vi "Sort References By Type.vi"(10 "Controls[]":refnum<vi>[](array[refnum])) -> (2 "Controls":T1)   [LabVIEW 2015, in "AutoRegistration.lvlib" / "AbstractAutoRegistration.lvclass"]
uses:
  AbstractAutoRegistration.lvclass
  Registration References.ctl
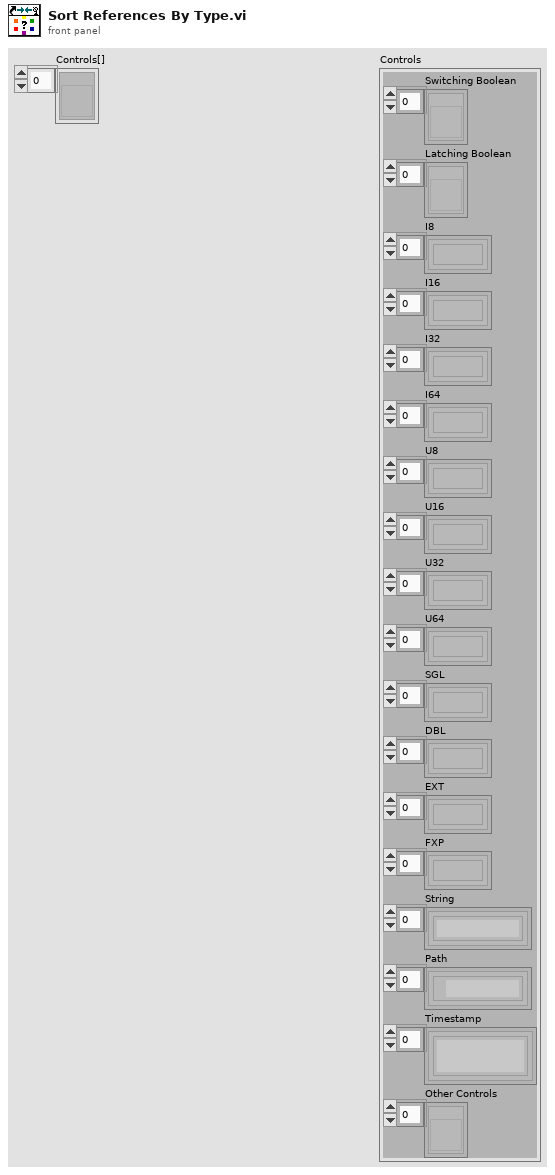
[diagram p1: front panel]
types:
  T1 = typedef "AutoRegistration.lvlib/AbstractAutoRegistration.lvclass/Registration References.ctl" = cluster{"Switching Boolean":refnum<vi>[], "Latching Boolean":refnum<vi>[], "I8":refnum<vi>[], "I16":refnum<vi>[], "I32":refnum<vi>[], "I64":refnum<vi>[], "U8":refnum<vi>[], "U16":refnum<vi>[], "U32":refnum<vi>[], "U64":refnum<vi>[], "SGL":refnum<vi>[], "DBL":refnum<vi>[], "EXT":refnum<vi>[], "FXP":refnum<vi>[], "String":refnum<vi>[], "Path":refnum<vi>[], "Timestamp":refnum<vi>[], "Other Controls":refnum<vi>[]}
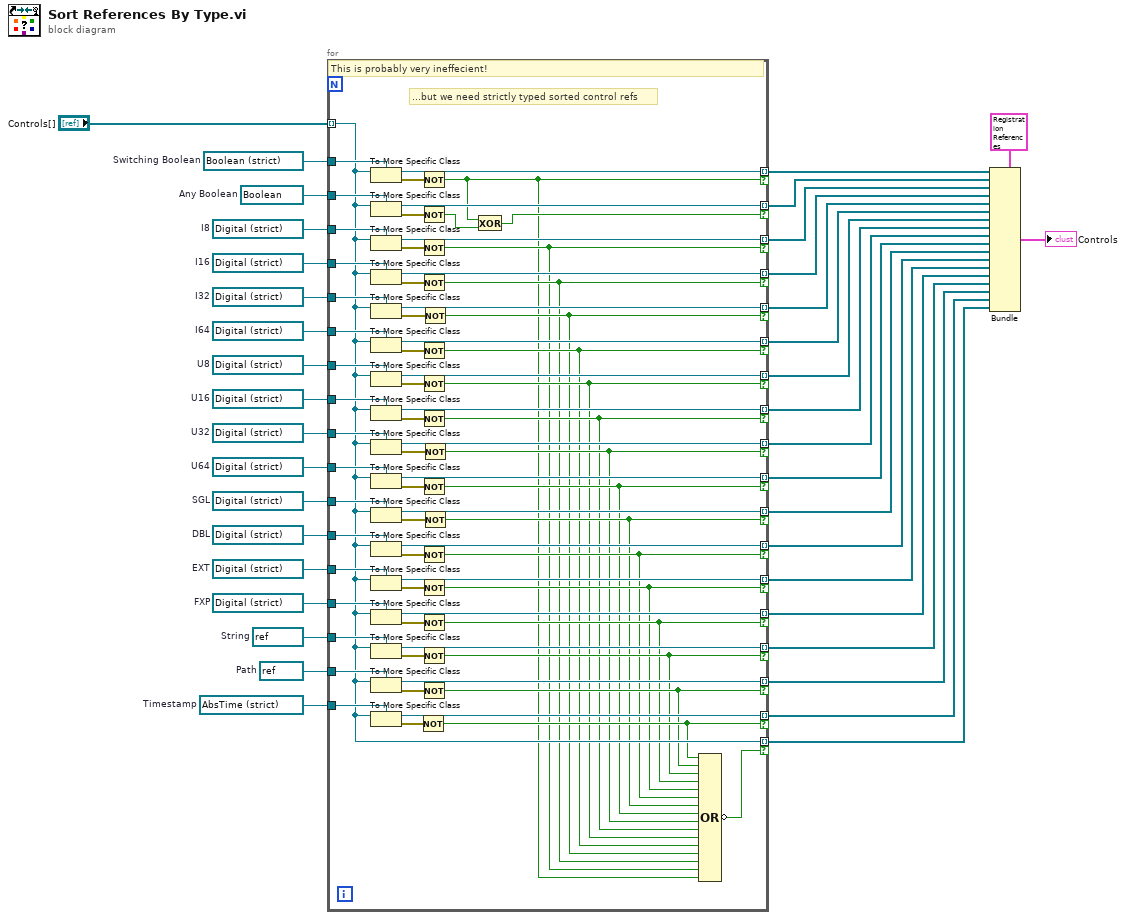
[diagram p0: block diagram]
diagram:
  w21 = refnum<vi> refnum  # Switching Boolean
  w22 = refnum<vi> refnum  # Any Boolean
  w23 = refnum<vi> refnum  # I8
  w24 = refnum<vi> refnum  # I16
  w25 = refnum<vi> refnum  # I32
  w26 = refnum<vi> refnum  # I64
  w27 = refnum<vi> refnum  # U8
  w28 = refnum<vi> refnum  # U16
  w29 = refnum<vi> refnum  # U32
  w30 = refnum<vi> refnum  # U64
  w31 = refnum<vi> refnum  # SGL
  w32 = refnum<vi> refnum  # DBL
  w33 = refnum<vi> refnum  # EXT
  w34 = refnum<vi> refnum  # FXP
  w35 = refnum<vi> refnum  # String
  w36 = refnum<vi> refnum  # Path
  w37 = refnum<vi> refnum  # Timestamp
  n1 = for {
    tunnel: "Controls[]" -> [w56] mode=indexing
    tunnel: w37 -> [w109]
    tunnel: w36 -> [w108]
    tunnel: w35 -> [w107]
    tunnel: w34 -> [w106]
    tunnel: w33 -> [w105]
    tunnel: w32 -> [w104]
    tunnel: w31 -> [w103]
    tunnel: w30 -> [w102]
    tunnel: w29 -> [w101]
    tunnel: w28 -> [w100]
    tunnel: w27 -> [w99]
    tunnel: w26 -> [w98]
    tunnel: w25 -> [w97]
    tunnel: w24 -> [w96]
    tunnel: w23 -> [w95]
    tunnel: w22 -> [w94]
    tunnel: w21 -> [w93]
    tunnel: [w92] -> w20 mode=indexing if=w39
    tunnel: [w91] -> w19 mode=indexing if=w57
    tunnel: [w90] -> w18 mode=indexing if=w40
    tunnel: [w89] -> w17 mode=indexing if=w41
    tunnel: [w88] -> w16 mode=indexing if=w42
    tunnel: [w87] -> w15 mode=indexing if=w43
    tunnel: [w86] -> w14 mode=indexing if=w44
    tunnel: [w85] -> w13 mode=indexing if=w45
    tunnel: [w84] -> w12 mode=indexing if=w46
    tunnel: [w83] -> w11 mode=indexing if=w47
    tunnel: [w82] -> w10 mode=indexing if=w48
    tunnel: [w81] -> w9 mode=indexing if=w49
    tunnel: [w80] -> w8 mode=indexing if=w50
    tunnel: [w79] -> w7 mode=indexing if=w51
    tunnel: [w78] -> w6 mode=indexing if=w52
    tunnel: [w77] -> w5 mode=indexing if=w53
    tunnel: [w76] -> w4 mode=indexing if=w54
    tunnel: [w56] -> w3 mode=indexing if=w55
    # "...but we need strictly typed sorted control refs"
    # "This is probably very ineffecient!"
    n2 = To More Specific Class(target class=w93, reference=w56) -> (specific class reference=w92:refnum<vi>, error out=w75:errorcluster)  [unwired: 1 in]
    n3 = To More Specific Class(target class=w94, reference=w56) -> (specific class reference=w91:refnum<vi>, error out=w74:errorcluster)  [unwired: 1 in]
    n4 = To More Specific Class(target class=w95, reference=w56) -> (specific class reference=w90:refnum<vi>, error out=w73:errorcluster)  [unwired: 1 in]
    n5 = To More Specific Class(target class=w96, reference=w56) -> (specific class reference=w89:refnum<vi>, error out=w72:errorcluster)  [unwired: 1 in]
    n6 = To More Specific Class(target class=w97, reference=w56) -> (specific class reference=w88:refnum<vi>, error out=w71:errorcluster)  [unwired: 1 in]
    n7 = To More Specific Class(target class=w98, reference=w56) -> (specific class reference=w87:refnum<vi>, error out=w70:errorcluster)  [unwired: 1 in]
    n8 = To More Specific Class(target class=w99, reference=w56) -> (specific class reference=w86:refnum<vi>, error out=w69:errorcluster)  [unwired: 1 in]
    n9 = To More Specific Class(target class=w100, reference=w56) -> (specific class reference=w85:refnum<vi>, error out=w68:errorcluster)  [unwired: 1 in]
    n10 = To More Specific Class(target class=w101, reference=w56) -> (specific class reference=w84:refnum<vi>, error out=w67:errorcluster)  [unwired: 1 in]
    n11 = To More Specific Class(target class=w102, reference=w56) -> (specific class reference=w83:refnum<vi>, error out=w66:errorcluster)  [unwired: 1 in]
    n12 = To More Specific Class(target class=w103, reference=w56) -> (specific class reference=w82:refnum<vi>, error out=w65:errorcluster)  [unwired: 1 in]
    n13 = To More Specific Class(target class=w104, reference=w56) -> (specific class reference=w81:refnum<vi>, error out=w64:errorcluster)  [unwired: 1 in]
    n14 = To More Specific Class(target class=w105, reference=w56) -> (specific class reference=w80:refnum<vi>, error out=w63:errorcluster)  [unwired: 1 in]
    n15 = To More Specific Class(target class=w106, reference=w56) -> (specific class reference=w79:refnum<vi>, error out=w62:errorcluster)  [unwired: 1 in]
    n16 = To More Specific Class(target class=w107, reference=w56) -> (specific class reference=w78:refnum<vi>, error out=w61:errorcluster)  [unwired: 1 in]
    n17 = To More Specific Class(target class=w108, reference=w56) -> (specific class reference=w77:refnum<vi>, error out=w60:errorcluster)  [unwired: 1 in]
    n18 = To More Specific Class(target class=w109, reference=w56) -> (specific class reference=w76:refnum<vi>, error out=w59:errorcluster)  [unwired: 1 in]
    n19 = Not(x=w59) -> (.not. x?=w54:bool)
    n20 = Not(x=w75) -> (.not. x?=w39:bool)
    n21 = Not(x=w74) -> (.not. x?=w58:bool)
    n22 = Not(x=w73) -> (.not. x?=w40:bool)
    n23 = Not(x=w72) -> (.not. x?=w41:bool)
    n24 = Not(x=w70) -> (.not. x?=w43:bool)
    n25 = Not(x=w69) -> (.not. x?=w44:bool)
    n26 = Not(x=w68) -> (.not. x?=w45:bool)
    n27 = Not(x=w66) -> (.not. x?=w47:bool)
    n28 = Not(x=w64) -> (.not. x?=w49:bool)
    n29 = Not(x=w63) -> (.not. x?=w50:bool)
    n30 = Not(x=w62) -> (.not. x?=w51:bool)
    n31 = Not(x=w61) -> (.not. x?=w52:bool)
    n32 = Not(x=w60) -> (.not. x?=w53:bool)
    n33 = Not(x=w71) -> (.not. x?=w42:bool)
    n34 = Not(x=w67) -> (.not. x?=w46:bool)
    n35 = Not(x=w65) -> (.not. x?=w48:bool)
    n36 = Exclusive Or(1:w58, 2:w39) -> (0:w57:bool)
    n37 = Compound Arithmetic op=OR(w54, w53, w52, w51, w50, w49, w48, w47, w46, w45, w44, w43, w42, w41, w40, w39) -> (invert w55:bool)
  }
  n38 = Bundle(cluster=T1 {"Switching Boolean"=[], "Latching Boolean"=[], "I8"=[], "I16"=[], "I32"=[], "I64"=[], "U8"=[], "U16"=[], "U32"=[], "U64"=[], "SGL"=[], "DBL"=[], "EXT"=[], "FXP"=[], "String"=[], "Path"=[], "Timestamp"=[], "Other Controls"=[]} ("Controls"), "Switching Boolean"=w20, "Latching Boolean"=w19, "I8"=w18, "I16"=w17, "I32"=w16, "I64"=w15, "U8"=w14, "U16"=w13, "U32"=w12, "U64"=w11, "SGL"=w10, "DBL"=w9, "EXT"=w8, "FXP"=w7, "String"=w6, "Path"=w5, "Timestamp"=w4, "Other Controls"=w3) -> (→"Controls":T1)
